vi "sendAllMessages.vi"(8 "error in (no error)":errorcluster, 11 "TCPCommunicator in":refnum<class "TCPCommunicator.lvclass">) -> (0 "error out":errorcluster, 3 "TCPCommunicator out":refnum<class "TCPCommunicator.lvclass">)   [LabVIEW 2016, in "TCPCommunicator.lvclass"]
uses:
  TCPCommunicator.lvclass
  TCPCommunicator.lvclass/TCPCommunicator.ctl
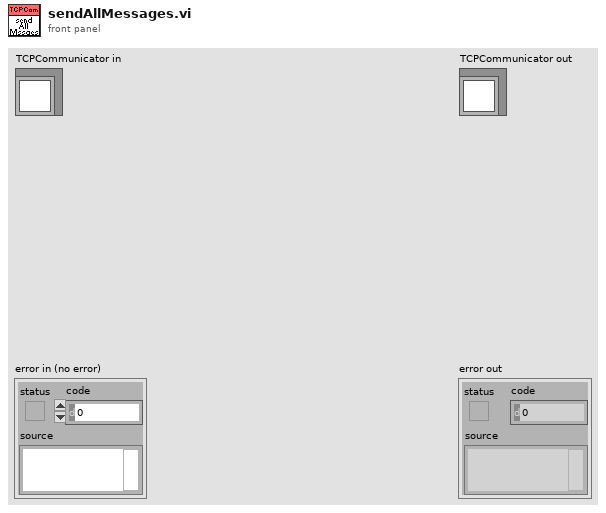
[diagram p1: front panel]
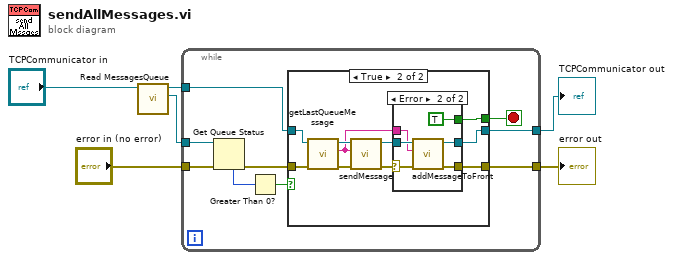
[diagram p0: block diagram]
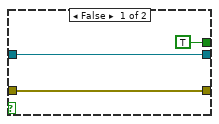
[diagram p2: hidden frame]
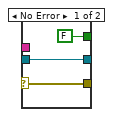
[diagram p3: hidden frame]
diagram:
  n1 = call "Read MessagesQueue.vi"("TCPCommunicator in"="TCPCommunicator in") -> ("MessagesQueue"=w5:refnum<queue>, "TCPCommunicator out"=w6:refnum<class "TCPCommunicator.lvclass">)  [unwired: 8 in, 1 out]
  n2 = while {
    tunnel: "error in (no error)" -> [w14]
    tunnel: [w13] -> w3
    tunnel: w5 -> [w9]
    tunnel: w6 -> [w8]
    tunnel: [w7] -> w1
    stop <- w10 stop-if-true
    n3 = Get Queue Status(queue=w9, error in (no error)=w14) -> (error out=w15:errorcluster, # elements in queue=w12:i32)  [unwired: 1 in, 6 out]
    n4 = Greater Than 0?(x=w12) -> (x > 0?=w11:bool)
    n5 = case shown="True" w11 {
      tunnel: w15 -> [w18 w28]
      tunnel: [w18 w25] -> w13
      tunnel: [TRUE w26] -> w10
      tunnel: w8 -> [w16 w27]
      tunnel: [w16 w24] -> w7
      frame False {
      }
      frame True {
        n6 = call "getLastQueueMessage.vi"("error in (no error)"=w28, "TCPCommunicator in"=w27) -> ("error out"=w23:errorcluster, "lastMessage"=w21:string, "TCPCommunicator out"=w22:refnum<class "TCPCommunicator.lvclass">)  [unwired: 6 in, 1 out]
        n7 = call-dynamic "sendMessage.vi"("error in (no error)"=w23, "String"=w21, "TCPCommunicator in"=w22) -> ("error out"=w19:errorcluster, "TCPCommunicator out"=w20:refnum<class "TCPCommunicator.lvclass">)  [unwired: 7 in]
        n8 = case shown="Error" w19 {
          selector: w19 -> [w30 w34]
          tunnel: [FALSE TRUE] -> w26
          tunnel: [w30 w33] -> w25
          tunnel: w20 -> [w29 w36]
          tunnel: w21 -> [_ w35]
          tunnel: [w29 w32] -> w24
          frame No Error {
          }
          frame Error {
            n9 = call "addMessageToFront.vi"("error in (no error)"=w34, "message"=w35, "TCPCommunicator in"=w36) -> ("error out"=w33:errorcluster, "TCPCommunicator out"=w32:refnum<class "TCPCommunicator.lvclass">)  [unwired: 6 in, 1 out]
          }
        }
      }
    }
  }
  "error out" <- w3
  "TCPCommunicator out" <- w1
